vi "From Serial Form.vi"(6 "Serial Version":T1, 10 "Deserializer in":refnum<class "Deserializer.lvclass">, 11 "cCRDS in":refnum<class "cCRDS.lvclass">) -> (0 "error out":errorcluster, 2 "Deserializer out":refnum<class "Deserializer.lvclass">, 3 "cCRDS out":refnum<class "cCRDS.lvclass">)   [LabVIEW 2012]
uses:
  <userlib>/Serialization/Serializable/Serializable.lvclass
  Reusable/Serial IO/Serial IO.lvclass
  <userlib>/Serialization/Serializable/Remove Serializable.vi
  Data/cCRDS Data.lvclass
  cCRDS.lvclass
  <userlib>/Serialization/Serializable/Remove Single.vi
  <userlib>/Serialization/Serializable/Remove Boolean.vi
  Reusable/CRDS/Data/Main/CRDS Data.lvclass
  <userlib>/Serialization/Serialization Common/Serial Version.ctl
  <userlib>/Serialization/Serialization Common/Serialization Common.lvlib
  <userlib>/Serialization/Deserializer/Deserializer.lvclass
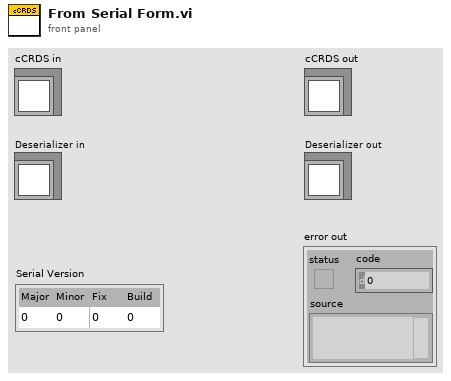
[diagram p1: front panel]
types:
  T1 = typedef "Serialization Common.lvlib/Serial Version.ctl" = cluster{"Major":u16, "Minor":u16, "Fix":u16, "Build":u16}
  T2 = cluster{cluster{"[0]":sgl, "[1]":sgl, "[2]":sgl}, "Numeric":sgl, "Numeric":sgl}
  T3 = cluster{cluster{cluster{"[0]":sgl, "[1]":sgl, "[2]":sgl}, "Numeric":sgl, "Numeric":sgl}, cluster{cluster{"[0]":sgl, "[1]":sgl, "[2]":sgl}, "Numeric":sgl, "Numeric":sgl}}
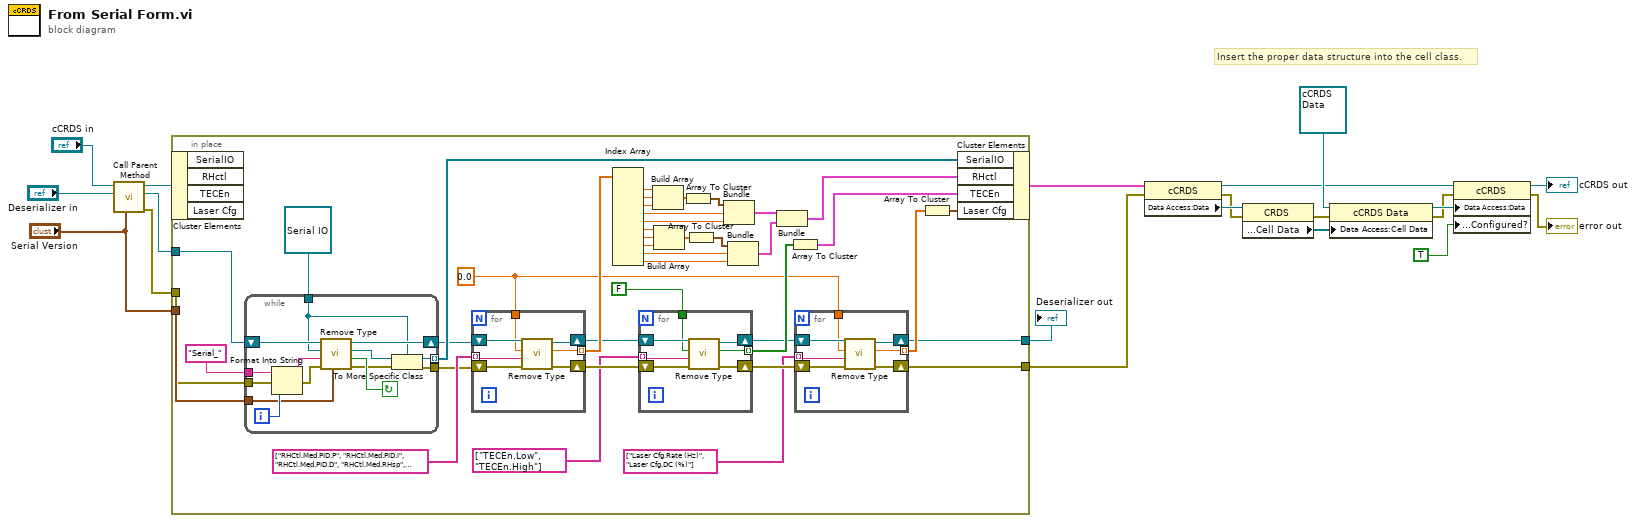
[diagram p0: block diagram]
diagram:
  # "Insert the proper data structure into the cell class."
  n1 = call-parent "Call Parent Method"("Serial Version"="Serial Version", "Deserializer in"="Deserializer in", "Instrument in"="cCRDS in") -> ("error out"=w15:errorcluster, "Deserializer out"=w17:refnum<class "Deserializer.lvclass">, "Instrument out"=w18:refnum<class "cCRDS.lvclass">)  [unwired: 6 in]
  n2 = in-place {
    in-place-border: w17 -> [w60]
    in-place-border: "Serial Version" -> [w58]
    in-place-border: w15 -> [w56]
    in-place-border: [w23] -> w14
    in-place-border: [w21] -> w11
    w28 = sgl 0.0
    n3 = in-place-cluster #1(w18) -> ()  [unwired: 4 out]
    n4 = while {
      tunnel: refnum<class "Serial IO.lvclass"> refnum ("Serial IO.lvclass") -> [w89]
      tunnel: [w87] -> w53
      tunnel: [w86] -> w59 mode=indexing
      tunnel: w58 -> [w85]
      tunnel: "Serial_" ("initial string") -> [w84]
      tunnel: w56 -> [w83]
      shift-right: [w91] -> w54
      shift-left: w60 -> [w96]
      i -> [w95]
      stop <- w92 continue-if-true
      n5 = Format Into String(initial string=w84, error in=w83, w95) -> (resulting string=w93:string, error out=w94:errorcluster)  [unwired: 1 in]
      n6 = call-poly <userlib>:"Remove Type.vi"("Serial Version"=w85, "error in (no error)"=w94, "Name"=w93, "Default Value"=w89, "Deserializer in"=w96) -> ("error out"=w88:errorcluster, "Found?"=w92:bool, "Serializable"=w90:refnum<class "Serializable.lvclass">, "Deserializer out"=w91:refnum<class "Deserializer.lvclass">)  [unwired: 3 in]
      n7 = To More Specific Class(target class=w89, reference=w90, error in=w88) -> (specific class reference=w86:refnum<class "Serial IO.lvclass">, error out=w87:errorcluster)
    }
    n8 = for {
      shift-right: [w81] -> w34
      shift-left: w54 -> [w82]
      tunnel: string[] ["RHCtl.Med.PID.P", "RHCtl.Med.PID.I", "RHCtl.Med.PID.D", "RHCtl.Med.RHsp", "RHCtl.Med.Tsp", "RHCtl.High.PID.P", "RHCtl.High.PID.I", "RHCtl.High.PID.D", "RHCtl.High.RHsp", "RHCtl.High.Tsp"] -> [w78] mode=indexing
      shift-right: [w80] -> w33
      shift-left: w53 -> [w79]
      tunnel: w28 -> [w77]
      tunnel: [w76] -> w52 mode=indexing
      n9 = call-poly <userlib>:"Remove Type.vi"("error in (no error)"=w79, "Name"=w78, "Default Value"=w77, "Deserializer in"=w82) -> ("error out"=w80:errorcluster, "Numeric"=w76:sgl, "Deserializer out"=w81:refnum<class "Deserializer.lvclass">)  [unwired: 4 in, 1 out]
    }
    n10 = Index Array(array=w52) -> (element #1=w51:sgl, element #2=w49:sgl, element #3=w50:sgl, element #4=w46:sgl, element #5=w45:sgl, element #6=w43:sgl, element #7=w42:sgl, element #8=w41:sgl, element #9=w39:sgl, element #10=w38:sgl)  [unwired: 10 in]
    n11 = for {
      shift-right: [w74] -> w27
      shift-left: w34 -> [w75]
      tunnel: string[] ["TECEn.Low", "TECEn.High"] -> [w71] mode=indexing
      shift-right: [w73] -> w26
      shift-left: w33 -> [w72]
      tunnel: FALSE -> [w70]
      tunnel: [w69] -> w30 mode=indexing
      n12 = call-poly <userlib>:"Remove Type.vi"("error in (no error)"=w72, "Name"=w71, "Default Value"=w70, "Deserializer in"=w75) -> ("error out"=w73:errorcluster, "Boolean"=w69:bool, "Deserializer out"=w74:refnum<class "Deserializer.lvclass">)  [unwired: 4 in, 1 out]
    }
    n13 = Build Array(w51, w49, w50) -> (w48:sgl[])
    n14 = Build Array(w43, w42, w41) -> (w44:sgl[])
    n15 = Array To Cluster(array=w48) -> (cluster=w47:cluster{"[0]":sgl, "[1]":sgl, "[2]":sgl})
    n16 = Array To Cluster(array=w44) -> (cluster=w40:cluster{"[0]":sgl, "[1]":sgl, "[2]":sgl})
    n17 = Bundle(w47, "Numeric"=w46, "Numeric"=w45) -> (w37:T2)  [unwired: 1 in]
    n18 = Bundle(w40, "Numeric"=w39, "Numeric"=w38) -> (w36:T2)  [unwired: 1 in]
    n19 = Bundle(w37, w36) -> (w35:T3)  [unwired: 1 in]
    n20 = Array To Cluster(array=w30) -> (cluster=w29:cluster{"[0]":bool, "[1]":bool})
    n21 = for {
      shift-right: [w67] -> w23
      shift-left: w27 -> [w68]
      tunnel: string[] ["Laser Cfg.Rate (Hz)", "Laser Cfg.DC (%)"] -> [w64] mode=indexing
      shift-right: [w66] -> w21
      shift-left: w26 -> [w65]
      tunnel: w28 -> [w63]
      tunnel: [w62] -> w24 mode=indexing
      n22 = call-poly <userlib>:"Remove Type.vi"("error in (no error)"=w65, "Name"=w64, "Default Value"=w63, "Deserializer in"=w68) -> ("error out"=w66:errorcluster, "Numeric"=w62:sgl, "Deserializer out"=w67:refnum<class "Deserializer.lvclass">)  [unwired: 4 in, 1 out]
    }
    n23 = Array To Cluster(array=w24) -> (cluster=w22:cluster{"[0]":sgl, "[1]":sgl})
    n24 = in-place-cluster #1("SerialIO"=w59, "RHctl"=w35, "TECEn"=w29, "Laser Cfg"=w22) -> (w13:cluster{})
  }
  "Deserializer out" <- w14
  n25 = property class="cCRDS"(reference=w13, error in=w11) -> (reference out=w6:refnum<class "cCRDS.lvclass">, error out=w7:errorcluster, "Data Access:Data"=w10:refnum<class "CRDS Data.lvclass">)
  n26 = property class="CRDS"(reference=w10, error in=w7) -> (error out=w8:errorcluster, "Data Access:Cell Data"=w9:refnum<class "CRDS Cell Data.lvclass">[])  [unwired: 1 out]
  n27 = property class="cCRDS Data"(reference=refnum<class "cCRDS Data.lvclass"> refnum ("cCRDS Data"), error in=w8, "Data Access:Cell Data"=w9) -> (reference out=w5:refnum<class "cCRDS Data.lvclass">, error out=w4:errorcluster)
  n28 = property class="cCRDS"(reference=w6, error in=w4, "Data Access:Data"=w5, "Data Access:Configured?"=TRUE ("Configured?")) -> (reference out=→"cCRDS out":refnum<class "cCRDS.lvclass">, error out=→"error out":errorcluster)
